vi "Start.vi"(8 "error in (no error)":errorcluster, 11 "DAQ in":refnum<class "DAQ.lvclass">) -> (3 "DAQ out":refnum<class "DAQ.lvclass">)   [LabVIEW 2019, in "DAQ.lvclass"]
uses:
  DAQ.lvclass
panel:
  out "error out":errorcluster
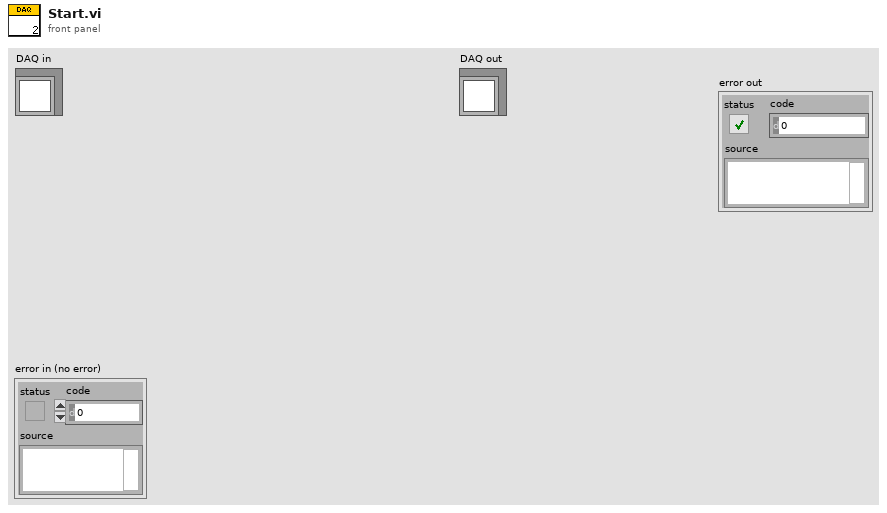
[diagram p1: front panel]
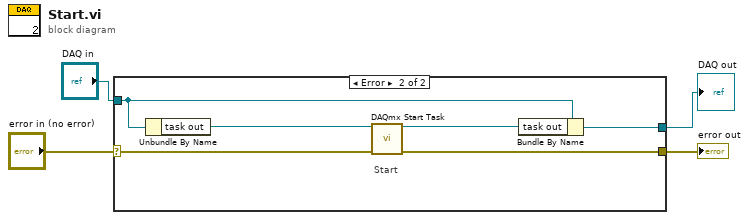
[diagram p0: block diagram]
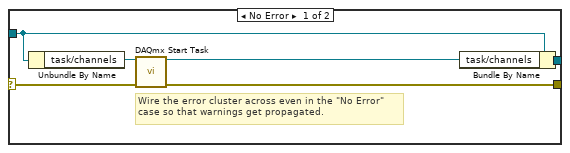
[diagram p2: hidden frame]
diagram:
  n1 = case shown="Error" "error in (no error)" {
    selector: "error in (no error)" -> [w10 w16]
    tunnel: [w9 w11] -> w1
    tunnel: "DAQ in" -> [w7 w13]
    tunnel: [w5 w12] -> w2
    frame No Error {
      # "Wire the error cluster across even in the \"No Error\"\ncase so that warnings get propagated."
      n2 = Unbundle By Name(w7) -> ("task/channels"=w8:refnum<k21>)
      n3 = call <vilib>:"DAQmx Start Task.vi"("task/channels in"=w8, "error in"=w10) -> ("task out"=w6:refnum<k21>, "error out"=w9:errorcluster)  [unwired: 12 in]
      n4 = Bundle By Name(cluster=w7, "task/channels"=w6) -> (w5:refnum<class "DAQ.lvclass">)
    }
    frame Error {
      # "Start"
      n5 = Unbundle By Name(w13) -> ("task out"=w15:refnum<k21>)
      n6 = call <vilib>:"DAQmx Start Task.vi"("task/channels in"=w15, "error in"=w16) -> ("task out"=w14:refnum<k21>, "error out"=w11:errorcluster)  [unwired: 12 in]
      n7 = Bundle By Name(cluster=w13, "task out"=w14) -> (w12:refnum<class "DAQ.lvclass">)
    }
  }
  "DAQ out" <- w2
  "error out" <- w1
